vi "MATLAB_SCRIPT_CONCAT_STRING.vi"(0 "FILENAME":string, 1 "COLOR_STR":string, 4 "Line Style":string(combo)="-", 5 "Fit polynomiales":bool, 6 "Marker Shape":string(combo)="*", 7 "Wait":i32=3 min=0 max=15 step=1, 8 "Polydegree Line Width":i32=2 min=0 max=15 step=1, 9 "PolyDegree":i32=3 min=0 max=69 step=1, 10 "Line Width":i32=1 min=0 max=15 step=1, 11 "Marker Size":i32=2 min=1 max=15 step=1) -> (2 "SCRIPT_STR":string[](array[string]))   [LabVIEW 2013]
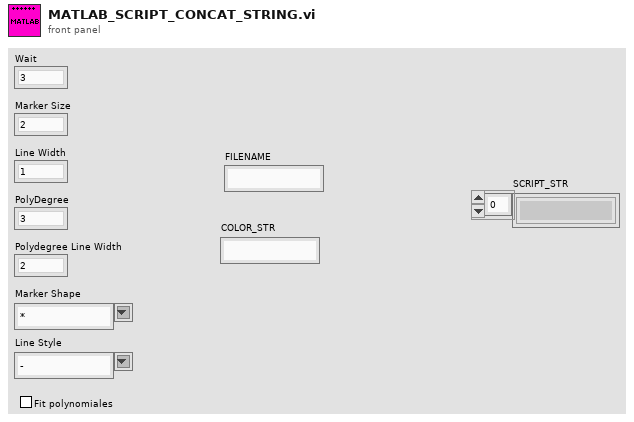
[diagram p1: front panel]
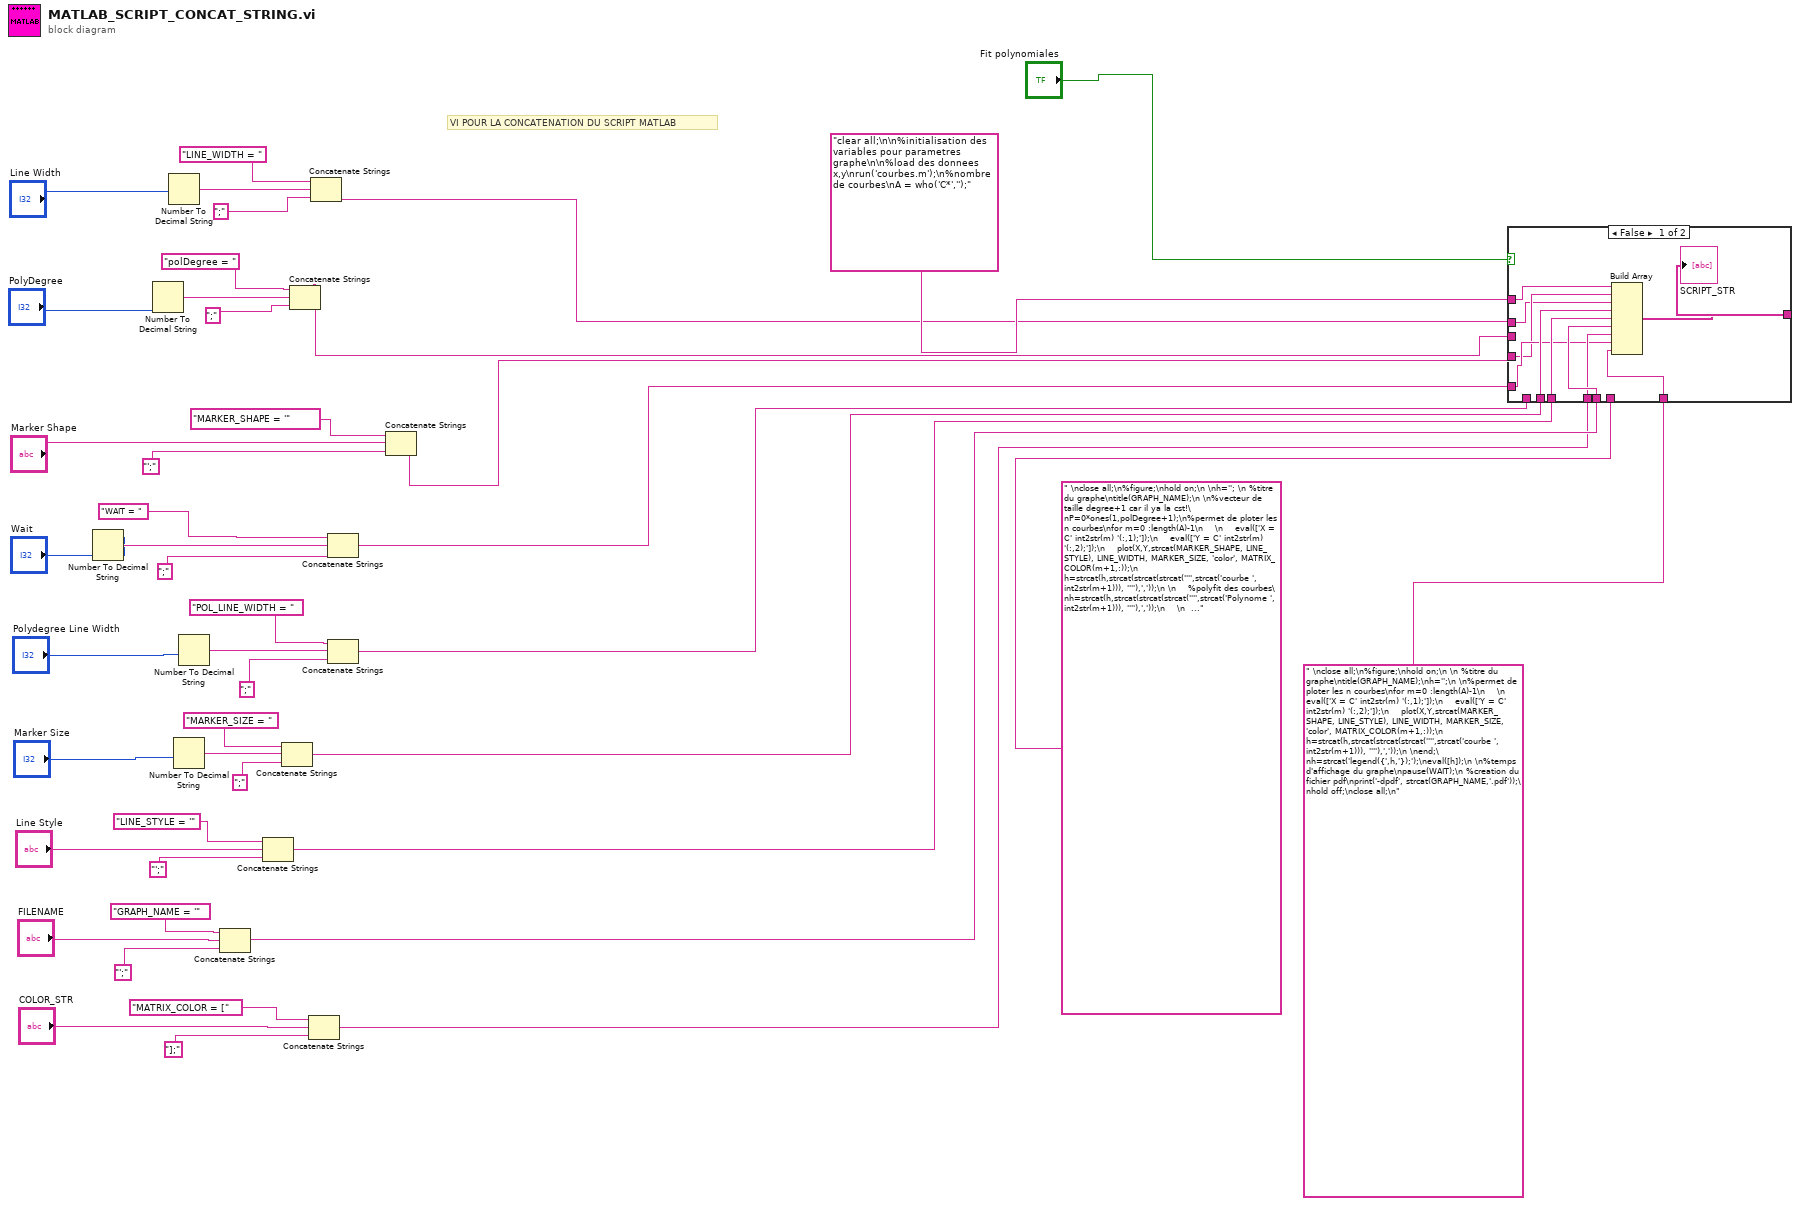
[diagram p0: block diagram]
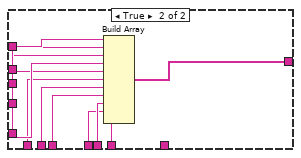
[diagram p2: hidden frame]
diagram:
  # "VI POUR LA CONCATENATION DU SCRIPT MATLAB"
  n1 = Number To Decimal String(number="Wait") -> (decimal integer string=w37:string)  [unwired: 1 in]
  n2 = Number To Decimal String(number="PolyDegree") -> (decimal integer string=w41:string)  [unwired: 1 in]
  n3 = Number To Decimal String(number="Line Width") -> (decimal integer string=w44:string)  [unwired: 1 in]
  n4 = Number To Decimal String(number="Marker Size") -> (decimal integer string=w29:string)  [unwired: 1 in]
  n5 = Number To Decimal String(number="Polydegree Line Width") -> (decimal integer string=w33:string)  [unwired: 1 in]
  n6 = Concatenate Strings("GRAPH_NAME = '", "FILENAME", "';") -> (w6:string)
  n7 = Concatenate Strings("LINE_STYLE = '", "Line Style", "';") -> (w7:string)
  n8 = Concatenate Strings("MARKER_SIZE = ", w29, ";") -> (w8:string)
  n9 = Concatenate Strings("polDegree = ", w41, ";") -> (w11:string)
  n10 = Concatenate Strings("MATRIX_COLOR = [" ("string"), "COLOR_STR", "];" ("string")) -> (w1:string)
  n11 = Concatenate Strings("LINE_WIDTH = ", w44, ";") -> (w12:string)
  n12 = Concatenate Strings("WAIT = ", w37, ";") -> (w4:string)
  n13 = Concatenate Strings("POL_LINE_WIDTH = ", w33, ";") -> (w9:string)
  n14 = Concatenate Strings("MARKER_SHAPE = '", "Marker Shape", "';") -> (w10:string)
  n15 = case shown="False" "Fit polynomiales" {
    tunnel: "clear all;\n\n%initialisation des variables pour parametres graphe\n\n%load des donnees x,y\nrun('courbes.m');\n%nombre de courbes\nA = who('C*','');" -> [w56 w68]
    tunnel: w12 -> [w47 w67]
    tunnel: w11 -> [_ w66]
    tunnel: w10 -> [w48 w65]
    tunnel: w4 -> [w49 w64]
    tunnel: w9 -> [_ w63]
    tunnel: w8 -> [w55 w62]
    tunnel: w7 -> [w54 w61]
    tunnel: w6 -> [w53 w60]
    tunnel: w1 -> [w51 w59]
    tunnel: " \nclose all;\n%figure;\nhold on;\n \nh=''; \n %titre du graphe\ntitle(GRAPH_NAME);\n \n%vecteur de taille degree+1 car il ya la cst!\nP=0*ones(1,polDegree+1);\n%permet de ploter les n courbes\nfor m=0 :length(A)-1\n    \n    eval(['X = C' int2str(m) '(:,1);']);\n    eval(['Y = C' int2str(m) '(:,2);']);\n    plot(X,Y,strcat(MARKER_SHAPE, LINE_STYLE), LINE_WIDTH, MARKER_SIZE, 'color', MATRIX_COLOR(m+1,:));\n   h=strcat(h,strcat(strcat(strcat('''',strcat('courbe ', int2str(m+1))), ''''),','));\n \n    %polyfit des courbes\nh=strcat(h,strcat(strcat(strcat('''',strcat('Polynome ', int2str(m+1))), ''''),','));\n    \n    P1= polyfit(X,Y,polDegree);\n    P(m+1,:)=P1;\n    plot(X,polyval(P1,X), strcat(MARKER_SHAPE, LINE_STYLE), POL_LINE_WIDTH, MARKER_SIZE, 'color', MATRIX_COLOR(m+1,:));\n    \nend;\nh=strcat('legend({',h,'});');\neval([h]);\n \n%temps d'affichage du graphe\npause(WAIT);\n %creation du fichier pdf\nprint('-dpdf', strcat(GRAPH_NAME,'.pdf'));\n%creation du fichier contenant les coefficient des polynomes\nxlswrite('P',P);\nhold off;\nclose all;\n" -> [_ w58]
    tunnel: " \nclose all;\n%figure;\nhold on;\n \n %titre du graphe\ntitle(GRAPH_NAME);\nh='';\n \n%permet de ploter les n courbes\nfor m=0 :length(A)-1\n    \n    eval(['X = C' int2str(m) '(:,1);']);\n    eval(['Y = C' int2str(m) '(:,2);']);\n    plot(X,Y,strcat(MARKER_SHAPE, LINE_STYLE), LINE_WIDTH, MARKER_SIZE, 'color', MATRIX_COLOR(m+1,:));\n   h=strcat(h,strcat(strcat(strcat('''',strcat('courbe ', int2str(m+1))), ''''),','));\n \nend;\nh=strcat('legend({',h,'});');\neval([h]);\n \n%temps d'affichage du graphe\npause(WAIT);\n %creation du fichier pdf\nprint('-dpdf', strcat(GRAPH_NAME,'.pdf'));\nhold off;\nclose all;\n" -> [w50 _]
    tunnel: [w52 w57] -> w2
    frame False {
      n16 = Build Array(w56, w48, w47, w55, w54, w53, w51, w49, w50) -> (w52:string[])
    }
    frame True {
      n17 = Build Array(w68, w67, w66, w65, w64, w63, w62, w61, w60, w59, w58) -> (w57:string[])
    }
  }
  "SCRIPT_STR" <- w2
